vi "Get Initial Info.vi"(11 "String":string="$AGENT.81,C8.C8,S*03") -> (2 "機種廠商代號":string, 3 "硬體版本":string)   [LabVIEW 2019]
panel:
  out "before substring":string
  in  "ToolString Input":string="$AGENT,53,VS-62U009+VS-69W014*71"
  out "after substring":string
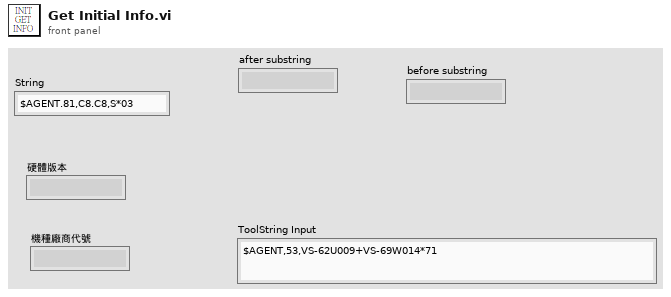
[diagram p1: front panel]
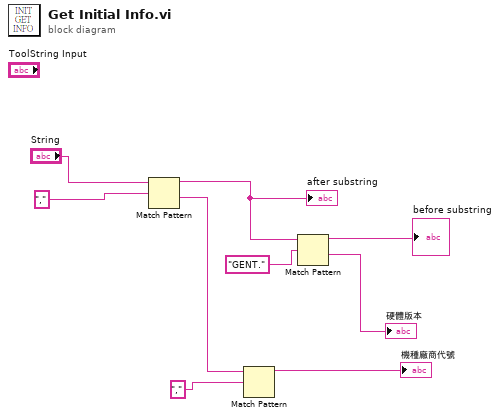
[diagram p0: block diagram]
diagram:
  n1 = Match Pattern(string="String", regular expression=",") -> (before substring=w5:string, after substring=w8:string)  [unwired: 1 in, 2 out]
  "after substring" <- w5
  n2 = Match Pattern(string=w8, regular expression=",") -> (before substring=→"機種廠商代號":string)  [unwired: 1 in, 3 out]
  n3 = Match Pattern(string=w5, regular expression="GENT.") -> (before substring=→"before substring":string, after substring=→"硬體版本":string)  [unwired: 1 in, 2 out]
